vi "_TangoGetAttributeInfo.vi"(2 "error in":errorcluster, 3 "attribute name":string, 4 "device name":string) -> (0 "error out":errorcluster, 1 "attribute info":T1={"device name"="", "attribute name"="", "r/w access"=enum."UNKNOWN_ACCESS_TYPE", "format"=enum."UNKNOWN_FORMAT", "data type"=enum."UNKNOW_DATA_TYPE", "level"=enum."UNKNOWN_LEVEL", "label"="", "unit"="", "display format"="", "min value"="", "max value"="", "min alarm"="", "max alarm"=""})   [LabVIEW 2014, in "tango.lvlib"]
uses:
  tango.lvlib
  Common VIs/Typedefs/_AttributeInfo_t.ctl
  Common VIs/Typedefs/_AttributeAccess_t.ctl
  Common VIs/Typedefs/_AttributeFormat_t.ctl
  Common VIs/Typedefs/_TangoDataType_t.ctl
  Common VIs/Typedefs/_AttributeLevel_t.ctl
  tango_binding.dll
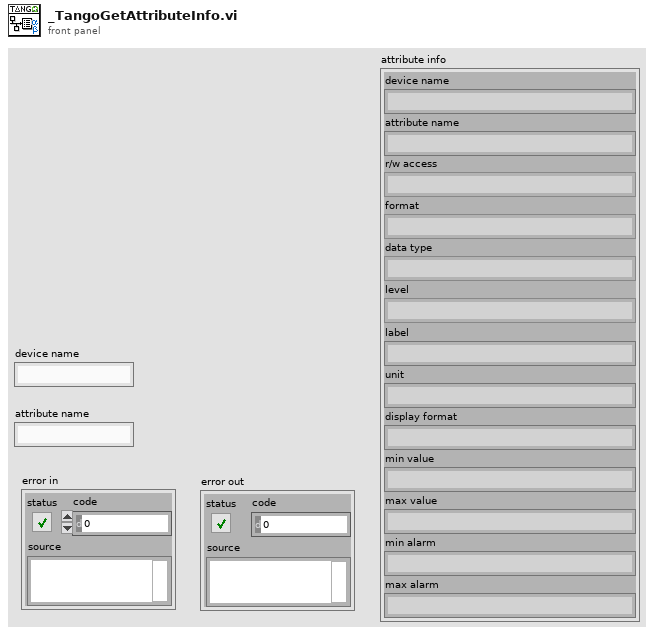
[diagram p1: front panel]
types:
  T1 = typedef "tango.lvlib/_AttributeInfo_t.ctl" = cluster{"device name":string, "attribute name":string, "r/w access":T2, "format":T3, "data type":T4, "level":T5, "label":string, "unit":string, "display format":string, "min value":string, "max value":string, "min alarm":string, "max alarm":string}
  T2 = typedef "tango.lvlib/_AttributeAccess_t.ctl" = enum16{"READ", "READ_WITH_WRITE", "WRITE", "READ_WRITE", "UNKNOWN_ACCESS_TYPE"}
  T3 = typedef "tango.lvlib/_AttributeFormat_t.ctl" = enum16{"SCALAR", "SPECTRUM", "IMAGE", "UNKNOWN_FORMAT"}
  T4 = typedef "tango.lvlib/_TangoDataType_t.ctl" = enum16{"VOID", "BOOLEAN", "SHORT", "LONG", "FLOAT", "DOUBLE", "USHORT", "ULONG", "STRING", "CHAR_ARRAY", "SHORT_ARRAY", "LONG_ARRAY", "FLOAT_ARRAY", "DOUBLE_ARRAY", "USHORT_ARRAY", "ULONG_ARRAY", "STRING_ARRAY", "LONG_STRING_ARRAY", "DOUBLE_STRING_ARRAY", "STATE", "CONST_STRING", "BOOLEAN_ARRAY", "UCHAR", "LONG64", "ULONG64", "LONG64_ARRAY", "ULONG64_ARRAY", "INT (not supported)", "ENCODED (not supported)", "ENUM", "PIPE_BLOB (not supported)", "STATE_ARRAY", "UNKNOW_DATA_TYPE"}
  T5 = typedef "tango.lvlib/_AttributeLevel_t.ctl" = enum16{"OPERATOR", "EXPERT", "UNKNOWN_LEVEL"}
  T6 = cluster{"device name":string, "attribute name":string, "r/w access":i16, "format":i16, "data type":i16, "level":i16, "label":string, "unit":string, "display format":string, "min value":string, "max value":string, "min alarm":string, "max alarm":string}
  T7 = cluster{"device name":string, "attribute name":string, "r/w access":i16, "format":i16, "data type":i16, "level":i16, "label":string, "unit":string, "display format":string, "min value":string, "max value":string, "min alarm":string, "max alarm":string}[]
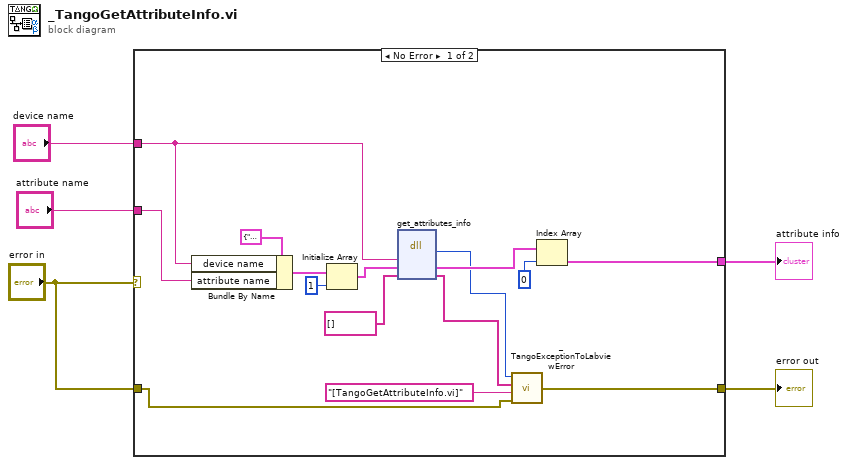
[diagram p0: block diagram]
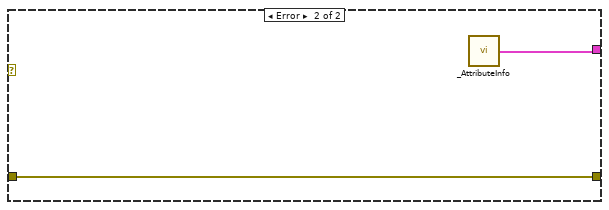
[diagram p2: hidden frame]
diagram:
  n1 = case shown="No Error" "error in" {
    tunnel: [w19 w22] -> w4
    tunnel: "error in" -> [w18 w22]
    tunnel: [w10 w21] -> w3
    tunnel: "device name" -> [w7 _]
    tunnel: "attribute name" -> [w6 _]
    frame No Error {
      n2 = Bundle By Name(cluster=T6 {"device name"="", "attribute name"="", "r/w access"=0, "format"=0, "data type"=0, "level"=0, "label"="", "unit"="", "display format"="", "min value"="", "max value"="", "min alarm"="", "max alarm"=""}, "device name"=w7, "attribute name"=w6) -> (w8:T6)
      n3 = Initialize Array(w8, 1 ("dimension size")) -> (w14:T7)
      n4 = dll-call lib="tango_binding.*" fn="get_attributes_info"("dev_name"=w7, "attrs_info_inout"=w14, "error_stack"=string[] [] ("error stack")) -> ("return type"=w11:i32, "attrs_info_inout"=w13:T7, "error_stack"=w12:string[])  [unwired: 4 in, 2 out]
      n5 = call "_TangoExceptionToLabviewError.vi"("error in"=w18, "location"="[TangoGetAttributeInfo.vi]", "error stack"=w12, "error code"=w11) -> ("error out"=w19:errorcluster)
      n6 = Index Array(array=w13, index=0 ("indice")) -> (element=w10:T6)
    }
    frame Error {
      n7 = call "_AttributeInfo.vi"() -> ("attribute info"=w21:T6)  [unwired: 15 in]
    }
  }
  "error out" <- w4
  "attribute info" <- w3
